vi "Str Array to String.vi"(11 "Array":string[](array[string])) -> (3 "String":string)   [LabVIEW 2022 SP3]
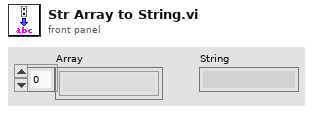
[diagram p1: front panel]
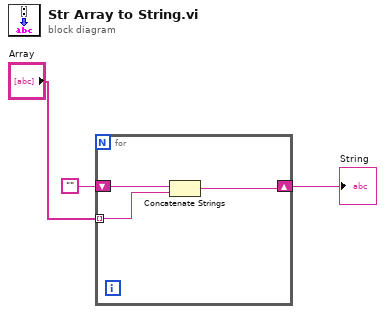
[diagram p0: block diagram]
diagram:
  n1 = for {
    tunnel: "Array" -> [w6] mode=indexing
    shift-right: [w5] -> w2
    shift-left: "" -> [w4]
    n2 = Concatenate Strings(w4, w6) -> (w5:string)
  }
  "String" <- w2
